vi "Get From Symbol Map New.vi"(8 "error in (no error)":errorcluster, 10 "Symbol Name":string, 11 "TwinCAT ADS in":refnum<class "TwinCAT ADS.lvclass">) -> (0 "error out":errorcluster, 1 ".NET Symbol Information":refnum<k24>, 2 "Found?":bool, 3 "TwinCAT ADS out":refnum<class "TwinCAT ADS.lvclass">)   [LabVIEW 2018, in "TwinCAT ADS.lvclass"]
uses:
  TwinCAT ADS.lvclass
  TwinCAT.Ads
  TwinCAT ADS.lvclass/TwinCAT ADS.ctl
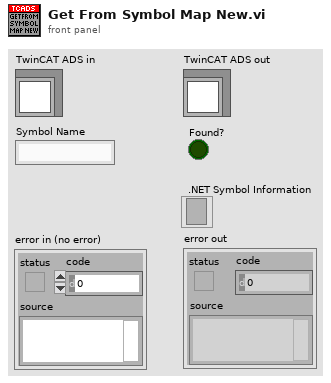
[diagram p1: front panel]
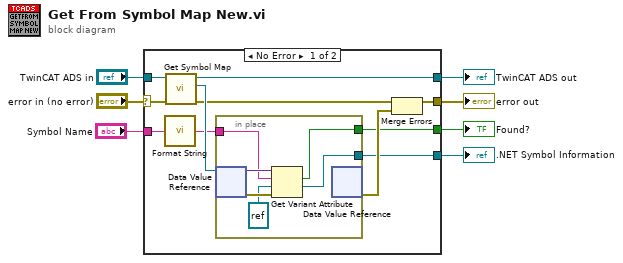
[diagram p0: block diagram]
diagram:
  n1 = case shown="No Error" "error in (no error)" {
    selector: "error in (no error)" -> [w11 w25]
    tunnel: "TwinCAT ADS in" -> [w17 w26]
    tunnel: "Symbol Name" -> [w15 _]
    tunnel: [w9 w25] -> w5
    tunnel: [w13 w26] -> w4
    tunnel: [w12 _] -> w2
    tunnel: [w8 _] -> w1
    frame No Error {
      n2 = call "Format String.vi"("String"=w15) -> ("Formated String"=w14:string)
      n3 = call "Get Symbol Map.vi"("error in (no error)"=w11, "TwinCAT ADS in"=w17) -> ("error out"=w10:errorcluster, "Symbol Map"=w16:refnum<data-value>, "TwinCAT ADS out"=w13:refnum<class "TwinCAT ADS.lvclass">)  [unwired: 7 in]
      n4 = in-place {
        in-place-border: w14 -> [w22]
        in-place-border: [w20] -> w8
        in-place-border: [w19] -> w12
        n5 = in-place-dvr #1(w16) -> (w23:variant, w24:errorcluster)
        n6 = Get Variant Attribute(Variant=w23, name=w22, default value (empty Variant)=refnum<k24> refnum (".NET Symbol Information"), error in=w24) -> (found=w19:bool, value=w20:refnum<k24>)  [unwired: 2 out]
        n7 = in-place-dvr #1() -> (w18:errorcluster)  [unwired: 1 in, 1 out]
      }
      n8 = Merge Errors(w10, w18) -> (w9:errorcluster)
    }
    frame Error {
    }
  }
  "error out" <- w5
  "TwinCAT ADS out" <- w4
  ".NET Symbol Information" <- w1
  "Found?" <- w2
